vi "Write All Dependencies Properties.vi"(8 "error in (no error)":errorcluster, 10 "All Dependencies Properties":T1[](array[typedef]), 11 "CustomDeviceRepo in":refnum<class "CustomDeviceRepo.lvclass">) -> (0 "error out":errorcluster, 3 "CustomDeviceRepo out":refnum<class "CustomDeviceRepo.lvclass">)   [LabVIEW 2019, in "CustomDeviceRepo.lvclass"]
uses:
  CustomDeviceRepo.lvclass
  XML Controls/Dependencies Properties.ctl
  XML Controls/Path Cluster.ctl
  XML Controls/Supported Targets.ctl
  CustomDeviceRepo.lvclass/CustomDeviceRepo.ctl
  VeriStand Custom Device XML Parser.lvlib
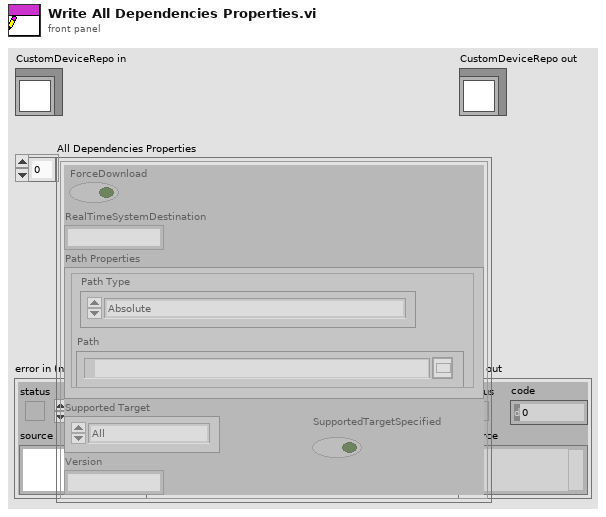
[diagram p1: front panel]
types:
  T1 = typedef "VeriStand Custom Device XML Parser.lvlib/Dependencies Properties.ctl" = cluster{"ForceDownload":bool, "RealTimeSystemDestination":string, "Path Properties":T2, "Supported Target":T3, "Version":string, "SupportedTargetSpecified":bool}
  T2 = typedef "VeriStand Custom Device XML Parser.lvlib/Path Cluster.ctl" = cluster{"Path":path, "Path Type":enum16{"Absolute", "To Base", "To Common Doc Dir", "To Application Data Dir"}}
  T3 = typedef "VeriStand Custom Device XML Parser.lvlib/Supported Targets.ctl" = enum16{"All", "Pharlap", "VxWorks", "Windows", "Linux_32_ARM", "Linux_x64", "PharlapWindows", "PharlapVxWorks", "VxWorksWindows"}
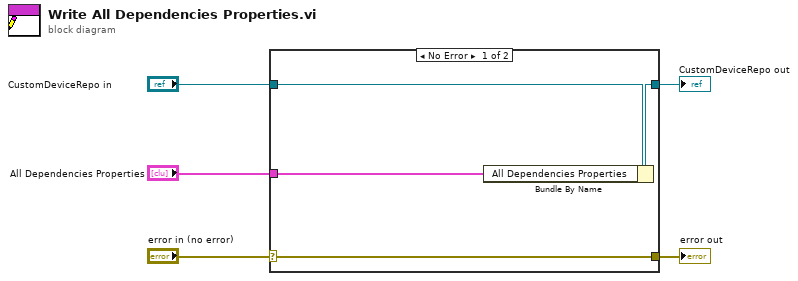
[diagram p0: block diagram]
diagram:
  n1 = case shown="No Error" "error in (no error)" {
    selector: "error in (no error)" -> [w9 w10]
    tunnel: [w9 w10] -> w4
    tunnel: [w7 w11] -> w2
    tunnel: "CustomDeviceRepo in" -> [w8 w11]
    tunnel: "All Dependencies Properties" -> [w6 _]
    frame No Error {
      n2 = Bundle By Name(cluster=w8, "All Dependencies Properties"=w6) -> (w7:refnum<class "CustomDeviceRepo.lvclass">)
    }
    frame Error {
    }
  }
  "error out" <- w4
  "CustomDeviceRepo out" <- w2
